vi "Calculate Number of Samples for Data Buffer.vi"(7 "Measurement":string, 10 "Sample rate":dbl, 11 "Number of samples":u32) -> (2 "Total no of samples per channel":u32)   [LabVIEW 2021]
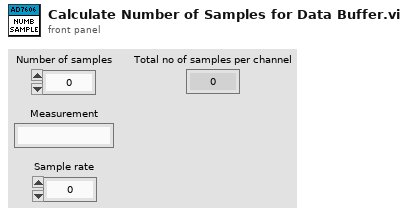
[diagram p1: front panel]
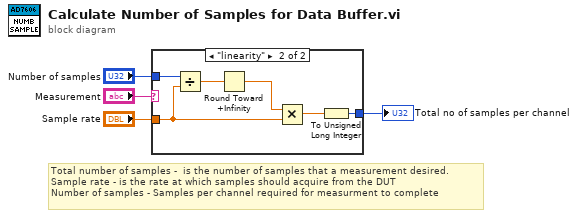
[diagram p0: block diagram]
diagram:
  # "Total number of samples -  is the number of samples that a measurement desired.\nSample rate - is the rate at which samples should acquire from the DUT\nNumber of samples - Samples per channel required for measurment to complete"
  n1 = case shown="\"linearity\"" "Measurement" {
    tunnel: [w5 w11] -> w4
    tunnel: "Sample rate" -> [_ w10]
    tunnel: "Number of samples" -> [w5 w9]
    frame Default {
    }
    frame "linearity" {
      n2 = Divide(x=w9, y=w10) -> (x/y=w8:dbl)
      n3 = Round Toward +Infinity(x=w8) -> (ceil(x): smallest int >= x=w7:dbl)
      n4 = Multiply(x=w7, y=w10) -> (x*y=w6:dbl)
      n5 = To Unsigned Long Integer(number=w6) -> (unsigned 32bit integer=w11:u32)
    }
  }
  "Total no of samples per channel" <- w4
